vi "Initialise.vi"(8 "error in (no error)":errorcluster, 10 "Message in":refnum<class "InitialiseMessage.lvclass">, 11 "DAQCascade512II in":refnum<class "DAQCascade512II.lvclass">) -> (0 "error out":errorcluster, 3 "DAQCascade512II out":refnum<class "DAQCascade512II.lvclass">)   [LabVIEW 2012, in "DAQCascade512II.lvclass"]
doc: "This method is called when an initialise message is received. It mainly initialises the RabbitMQ connectivity. \n\nOverride this method when your component needs special initialisation (e.g. of software or hardware resources). In that case, don't forget to call the parent for proper implementation. If your component owns subcomponents, they count as resources, so you have to initialise them by calling their own initialise functions"
uses:
  DAQCascade512II.lvclass
  <vilib>/Distrio/Murmex/InitialiseMessage/InitialiseMessage.lvclass
  <vilib>/Distrio/Murmex/Murmex/Murmex.lvclass
  DAQCascade512II.lvclass/DAQCascade512II.ctl
panel:
  out "intialized?":bool
  out "Camera\n Handle":u32
  # "This method is called when the INTIALISE\ntrigger is sent. \n\nOverride this method when your component needs to\nrespond to this trigger. \n\nCall parent for proper implementation"
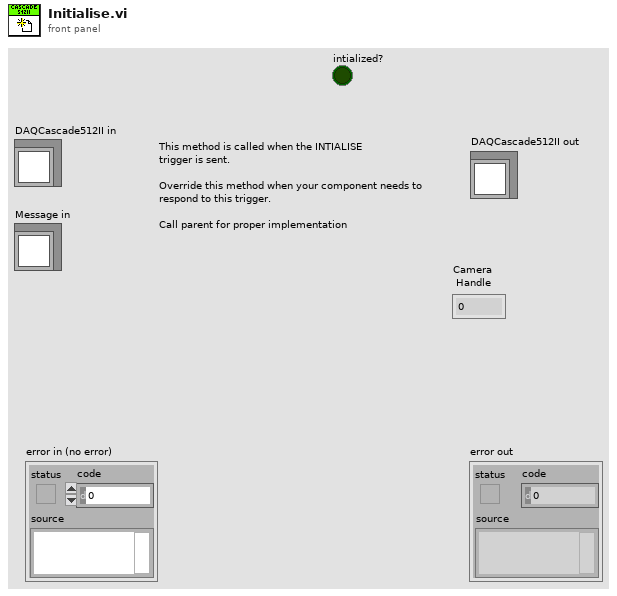
[diagram p1: front panel]
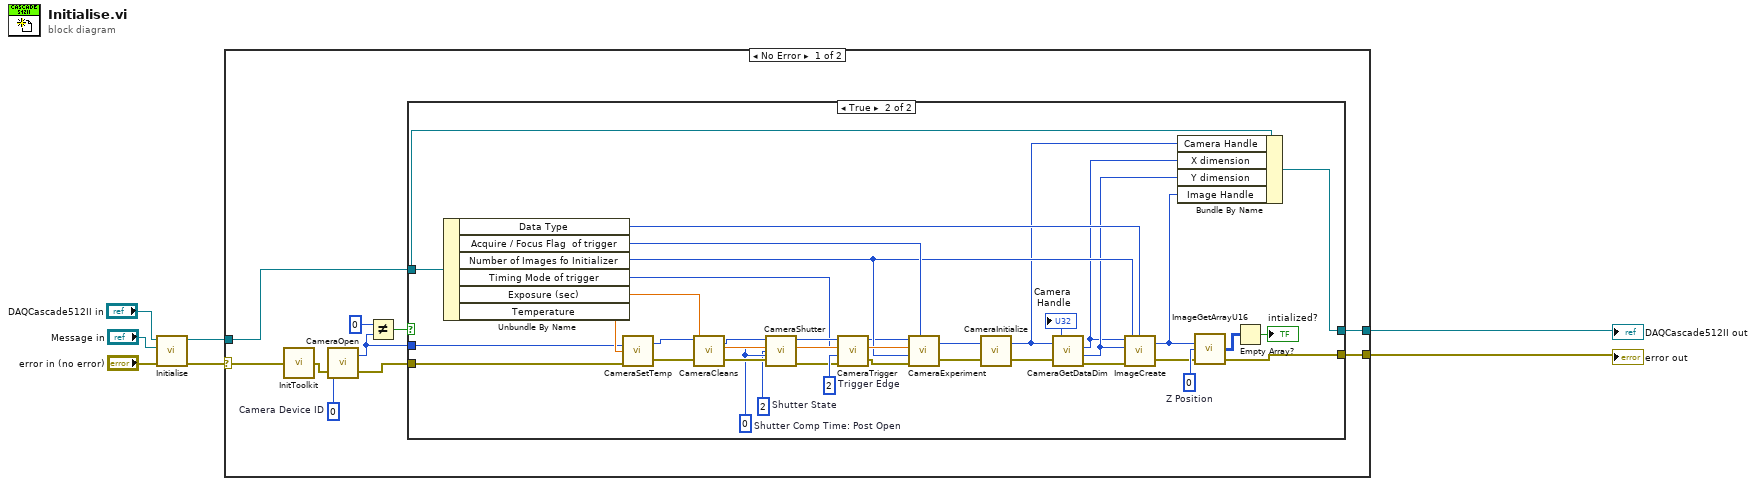
[diagram p0: block diagram]
diagram:
  n1 = call-parent "Initialise.vi"("error in (no error)"="error in (no error)", "Message in"="Message in", "Murmex in"="DAQCascade512II in") -> ("error out"=w4:errorcluster, "Murmex out"=w2:refnum<class "DAQCascade512II.lvclass">)  [unwired: 7 in]
  n2 = case shown="No Error" w4 {
    selector: w4 -> [w17 w56]
    tunnel: [w12 w56] -> w3
    tunnel: [w14 w55] -> w1
    tunnel: w2 -> [w13 w55]
    frame No Error {
      w16 = u32 0  # Camera Device ID
      n3 = call <userlib>:"InitToolkit.vi"("error in"=w17) -> ("error out"=w15:errorcluster)
      n4 = call <userlib>:"CameraOpen.vi"("error in"=w15, "Camera Device ID"=w16) -> ("error out"=w10:errorcluster, "Camera Handle"=w11:u32)
      n5 = Not Equal?(x=u32 0, y=w11) -> (x != y?=w8:bool)
      n6 = case shown="True" w8 {
        tunnel: w10 -> [w18 w54]
        tunnel: [w18 w22] -> w12
        tunnel: [w19 w44] -> w14
        tunnel: w11 -> [_ w43]
        tunnel: w13 -> [w19 w42]
        frame False {
        }
        frame True {
          w24 = u32 0  # Z Position
          w41 = u32 0  # Shutter Comp Time: Post Open
          w32 = u32 2  # Trigger Edge
          w26 = u32 2  # Shutter State
          n7 = Unbundle By Name(w42) -> ("Data Type"=w36:u32, "Acquire / Focus Flag  of trigger"=w46:u32, "Number of Images fo Initializer"=w39:u32, "Timing Mode of trigger"=w27:u32, "Exposure (sec)"=w45:dbl, "Temperature"=w47:dbl)
          n8 = call <userlib>:"CameraSetTemp.vi"("error in (no error)"=w54, "Temperature"=w47, "Camera Handle"=w43) -> ("error out"=w52:errorcluster, "Camera Handle"=w53:u32)
          n9 = call <userlib>:"CameraCleans.vi"("Camera Handle"=w53, "error in"=w52) -> ("Camera Handle"=w50:u32, "error out"=w51:errorcluster)  [unwired: 3 in]
          n10 = call <userlib>:"CameraShutter.vi"("Camera Handle"=w50, "Shutter Comp Time: Pre Open"=w41, "Shutter Comp Time: Post Open"=w41, "error in"=w51, "Shutter State"=w26) -> ("Camera Handle"=w31:u32, "error out"=w28:errorcluster)
          n11 = call <userlib>:"CameraTrigger.vi"("error in"=w28, "Trigger Edge"=w32, "Timing Mode"=w27, "Camera Handle"=w31) -> ("error out"=w29:errorcluster, "Camera Handle"=w30:u32)
          n12 = call <userlib>:"CameraExperiment.vi"("Acquire / Focus Flag"=w46, "error in"=w29, "Number of Images"=w39, "Exposure (sec)"=w45, "Camera Handle"=w30) -> ("error out"=w48:errorcluster, "Camera Handle"=w49:u32)  [unwired: 1 in]
          n13 = call <userlib>:"CameraInitialize.vi"("error in"=w48, "Camera Handle"=w49) -> ("error out"=w40:errorcluster, "Camera Handle"=w33:u32)
          n14 = call <userlib>:"CameraGetDataDim.vi"("Camera Handle"=w33, "error in"=w40) -> ("Camera Handle"=→"Camera\n Handle":u32, "Xdim"=w34:u32, "Ydim"=w35:u32, "error out"=w37:errorcluster)
          n15 = call <userlib>:"ImageCreate.vi"("X dimension"=w34, "Y dimension"=w35, "Data Type"=w36, "error in"=w37, "Number Of Frames"=w39) -> ("Image Handle"=w25:u32, "error out"=w23:errorcluster)
          n16 = Bundle By Name(cluster=w42, "Camera Handle"=w33, "X dimension"=w34, "Y dimension"=w35, "Image Handle"=w25) -> (w44:refnum<class "DAQCascade512II.lvclass">)
          n17 = call <userlib>:"ImageGetArrayU16.vi"("error in"=w23, "Z position"=w24, "Image Handle"=w25) -> ("error out"=w22:errorcluster, "Array uint 16"=w21:u16[][])  [unwired: 1 out]
          n18 = Empty Array?(array=w21) -> (empty?=→"intialized?":bool)
        }
      }
    }
    frame Error {
    }
  }
  "error out" <- w3
  "DAQCascade512II out" <- w1
